vi "control.vi"(10 "notifier in":refnum<notifier>) -> ()   [LabVIEW 2015]
doc: "execution of commands. here just various waits. go to stand by when finished."
uses:
  commands.ctl
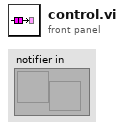
[diagram p1: front panel]
types:
  T1 = typedef "commands.ctl" = cluster{"command":enum16{"StandBy", "printHello", "printFRC", "printBalls", "exit"}, "data":variant}
  T2 = enum16{"StandBy", "printHello", "printFRC", "printBalls", "exit"}
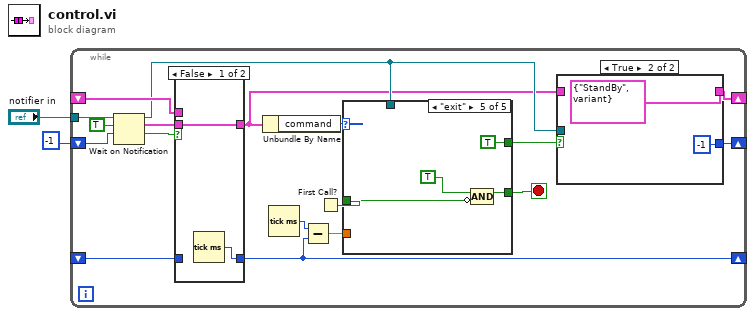
[diagram p0: block diagram]
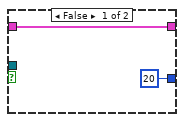
[diagram p2: hidden frame]
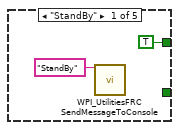
[diagram p4: hidden frame]
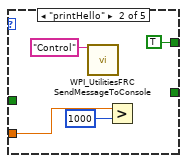
[diagram p5: hidden frame]
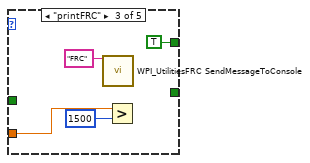
[diagram p6: hidden frame]
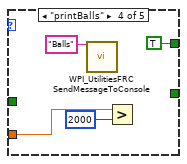
[diagram p7: hidden frame]
diagram:
  n1 = while {
    tunnel: "notifier in" -> [w20]
    shift-right: [w4] -> _
    shift-left: _ -> [w16]
    shift-right: [w12] -> _
    shift-left: _ -> [w15]
    shift-right: [w6] -> _
    shift-left: -1 ("timeout in ms (-1)") -> [w7]
    stop <- w19 stop-if-true
    n2 = Wait on Notification(notifier=w20, ignore previous (F)=TRUE, timeout in ms (-1)=w7) -> (notifier out=w9:refnum<notifier>, notification=w17:T1, timed out?=w18:bool)  [unwired: 1 in, 1 out]
    n3 = case shown="False" w18 {
      tunnel: w17 -> [w25 _]
      tunnel: w16 -> [_ w28]
      tunnel: [w25 w28] -> w3
      tunnel: w15 -> [_ w27]
      tunnel: [w26 w27] -> w12
      frame False {
        n4 = Tick Count (ms)() -> (millisecond timer value=w26:u32)
      }
      frame True {
      }
    }
    n5 = Unbundle By Name(w3) -> ("command"=w14:T2)
    n6 = Tick Count (ms)() -> (millisecond timer value=w13:u32)
    n7 = Subtract(x=w13, y=w12) -> (x-y=w11:dbl)
    n8 = First Call?() -> (First Call?: T/F=w8:bool)
    n9 = case shown="\"exit\"" w14 {
      tunnel: [_ _ _ _ w44] -> w19
      tunnel: w11 -> [_ w34 w38 w42 _]
      tunnel: [TRUE TRUE TRUE TRUE TRUE] -> w10
      tunnel: w9 -> [_ _ _ _ _]
      tunnel: w8 -> [_ _ _ _ w43]
      frame "StandBy" {
        n10 = call <vilib>:"WPI_UtilitiesFRC SendMessageToConsole.vi"("Message"="StandBy") -> ()  [unwired: 14 in, 1 out]
      }
      frame "printHello" {
        n11 = call <vilib>:"WPI_UtilitiesFRC SendMessageToConsole.vi"("Message"="Control") -> ()  [unwired: 14 in, 1 out]
        n12 = Greater?(x=w34, y=u32 1000) -> ()  [unwired: 1 out]
      }
      frame "printFRC" {
        n13 = call <vilib>:"WPI_UtilitiesFRC SendMessageToConsole.vi"("Message"="FRC") -> ()  [unwired: 14 in, 1 out]
        n14 = Greater?(x=w38, y=u32 1500) -> ()  [unwired: 1 out]
      }
      frame "printBalls" {
        n15 = call <vilib>:"WPI_UtilitiesFRC SendMessageToConsole.vi"("Message"="Balls") -> ()  [unwired: 14 in, 1 out]
        n16 = Greater?(x=w42, y=u32 2000) -> ()  [unwired: 1 out]
      }
      frame "exit" {
        n17 = Compound Arithmetic op=AND(TRUE, invert w43) -> (w44:bool)
      }
    }
    n18 = case shown="True" w10 {
      tunnel: w9 -> [_ _]
      tunnel: [20 -1] -> w6
      tunnel: [w21 T1 {"command"=enum."StandBy", "data"=variant}] -> w4
      tunnel: w3 -> [w21 _]
      frame False {
      }
      frame True {
      }
    }
  }
